vi "Create Sheep.vi"() -> (3 "Sheep.lvclass":refnum<class "Sheep.lvclass">)   [LabVIEW 2018, in "Sheep.lvclass"]
uses:
  Sheep.lvclass
  Sheep.lvclass/Sheep.ctl
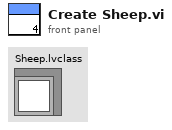
[diagram p1: front panel]
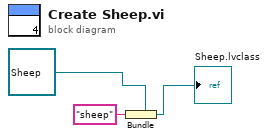
[diagram p0: block diagram]
diagram:
  n1 = Bundle(cluster=refnum<class "Sheep.lvclass"> refnum ("Sheep.lvclass"), "sheep" ("String")) -> (→"Sheep.lvclass":refnum<class "Sheep.lvclass">)
